vi "Build Mask.vi"(7 "Mask":T1, 8 "Error":errorcluster, 9 "Color":T2 {"Hue" scale=0.0..255.0 scale format="%#_3g"}, 11 "Cam Image":T1) -> (0 "Error Out":errorcluster, 3 "Mask Out":T1)   [LabVIEW 2017, in "VisionSystem.lvlib"]
uses:
  VisionSystem.lvlib
  Cluster_Threshold Settings.ctl
  <vilib>/vision/Image Controls.llb/IMAQ Image.ctl
  <vilib>/vision/NI_Vision_Development_Module.lvlib
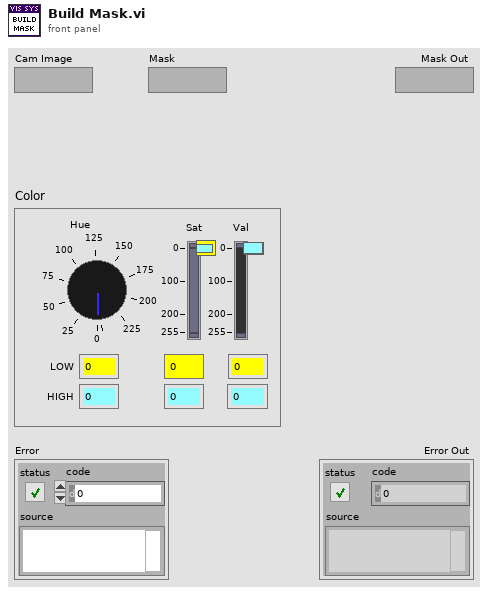
[diagram p1: front panel]
types:
  T1 = typedef "IMAQ Image.ctl" = refnum<image>
  T2 = typedef "VisionSystem.lvlib/Cluster_Threshold Settings.ctl" = cluster{"Hue":cluster{dbl, dbl}, "Sat":cluster{dbl, dbl}, "Val":cluster{dbl, dbl}}
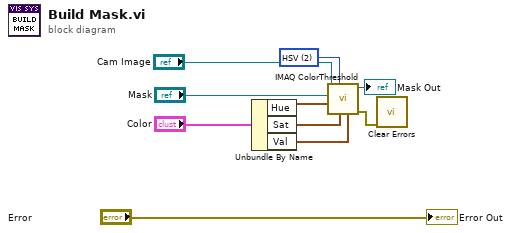
[diagram p0: block diagram]
diagram:
  w1 = u16 2 items=["RGB", "HSL", "HSV", "HSI"] ("Color Mode")
  n1 = Unbundle By Name("Color") -> ("Hue"=w7:cluster{dbl, dbl}, "Sat"=w6:cluster{dbl, dbl}, "Val"=w5:cluster{dbl, dbl})
  n2 = call "IMAQ ColorThreshold"("Blue or Luma or Val or Inten Range"=w5, "Green or Sat Range"=w6, "Color Mode"=w1, "Red or Hue Range"=w7, "Image Dst"="Mask", "Image Src"="Cam Image") -> ("error out"=w4:errorcluster, "Image Dst Out"=→"Mask Out":T1)  [unwired: 4 in]
  n3 = call <vilib>:"Clear Errors.vi"("error in (no error)"=w4) -> ()  [unwired: 5 in, 2 out]
  "Error Out" <- "Error"
